vi "Enqueue Message.vi"(6 "Priority Message? (F)":bool, 8 "error in (no error)":errorcluster, 10 "Element":T1) -> (0 "error out":errorcluster)   [LabVIEW 2020, in "Sensor Interface.lvlib"]
doc: "For a regular message, enqueue the message. For a priority message, enqueue it at the front of the queue."
uses:
  Sensor Interface.lvlib
  Private Controls/Message Cluster.ctl
  Private Controls/Message enum.ctl
  Private Controls/FG Actions.ctl
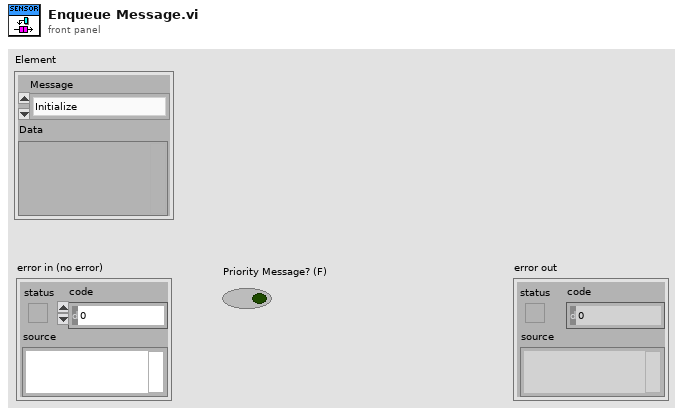
[diagram p1: front panel]
types:
  T1 = typedef "Sensor Interface.lvlib/Message Cluster.ctl" = cluster{"Message":T2, "Data":variant}
  T2 = typedef "Sensor Interface.lvlib/Message enum.ctl" = enum16{"Initialize", "State", "Error", "Exit"}
  T3 = typedef "Sensor Interface.lvlib/FG Actions.ctl" = enum16{"Get", "Set", "Clear"}
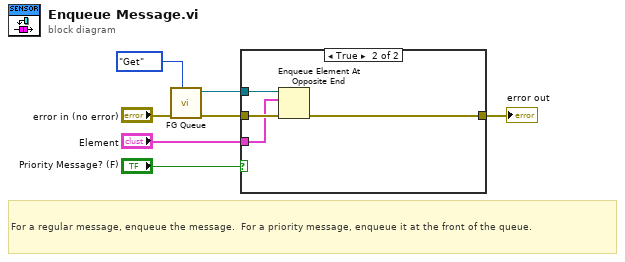
[diagram p0: block diagram]
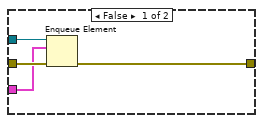
[diagram p2: hidden frame]
diagram:
  # "For a regular message, enqueue the message.  For a priority message, enqueue it at the front of the queue."
  n1 = call "FG Queue.vi"("FG Actions"=FG_Actions."Get", "error in (no error)"="error in (no error)") -> ("error out"=w4:errorcluster, "Message Queue Out"=w2:refnum<queue>)  [unwired: 8 in]
  n2 = case shown="True" "Priority Message? (F)" {
    tunnel: w4 -> [w11 w15]
    tunnel: [w10 w14] -> w6
    tunnel: w2 -> [w9 w13]
    tunnel: "Element" -> [w8 w12]
    frame False {
      n3 = Enqueue Element(queue=w9, element=w8, error in (no error)=w11) -> (error out=w10:errorcluster)  [unwired: 1 in, 2 out]
    }
    frame True {
      n4 = Enqueue Element At Opposite End(queue=w13, element=w12, error in (no error)=w15) -> (error out=w14:errorcluster)  [unwired: 1 in, 2 out]
    }
  }
  "error out" <- w6
